vi "Meca_Jocobian.vi"(0 "Joints":sgl[](array[numeric]), 1 "TRF_XYZ":sgl[](array[numeric])) -> (2 "J":dbl[][](array[numeric]), 3 "J-":dbl[][](array[numeric]), 4 "JT":dbl[][](array[numeric]), 5 "J-T":dbl[][](array[numeric]))   [LabVIEW 2018]
uses:
  <vilib>/Analysis/baseanly.llb/Real Inverse Matrix.vi
  <vilib>/Analysis/Matrix/Numeric/Conversions/Matrix To Array - RM.vi
  <vilib>/Analysis/NI_AALBase.lvlib
  <vilib>/Analysis/Matrix/NI_Matrix.lvlib
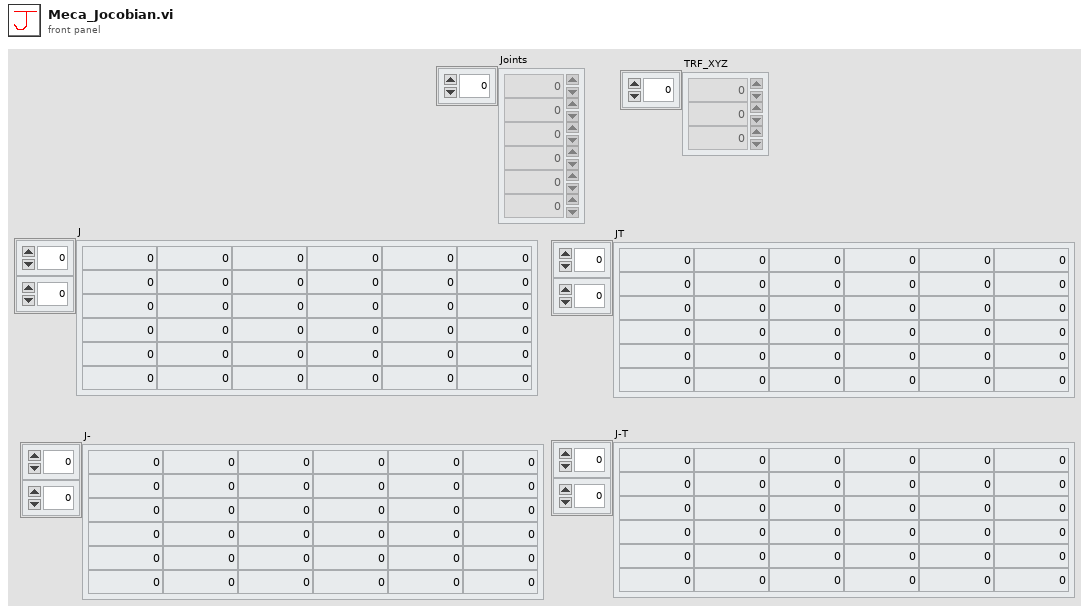
[diagram p1: front panel]
types:
  T1 = typedef "NI_Matrix.lvlib/RealMatrix.ctl" = dbl[][]
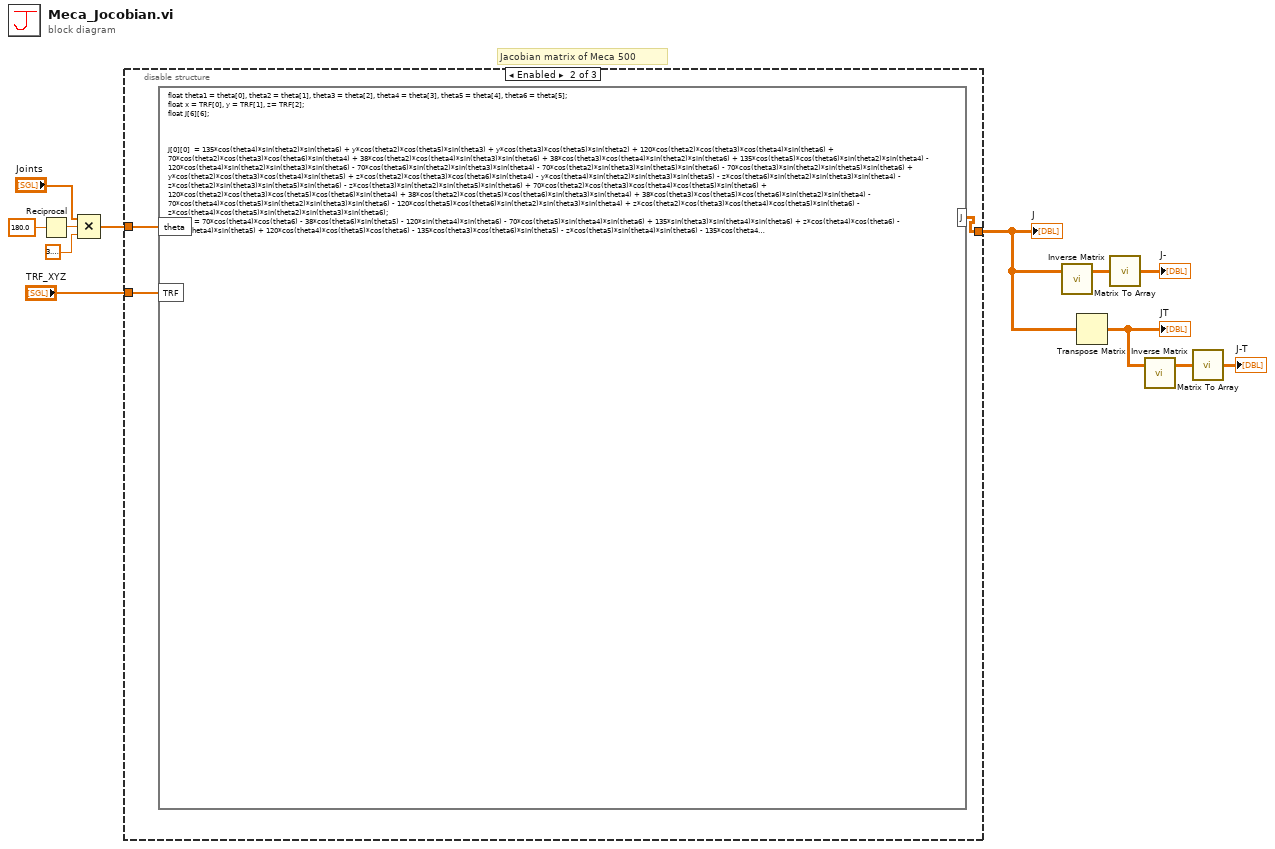
[diagram p0: block diagram]
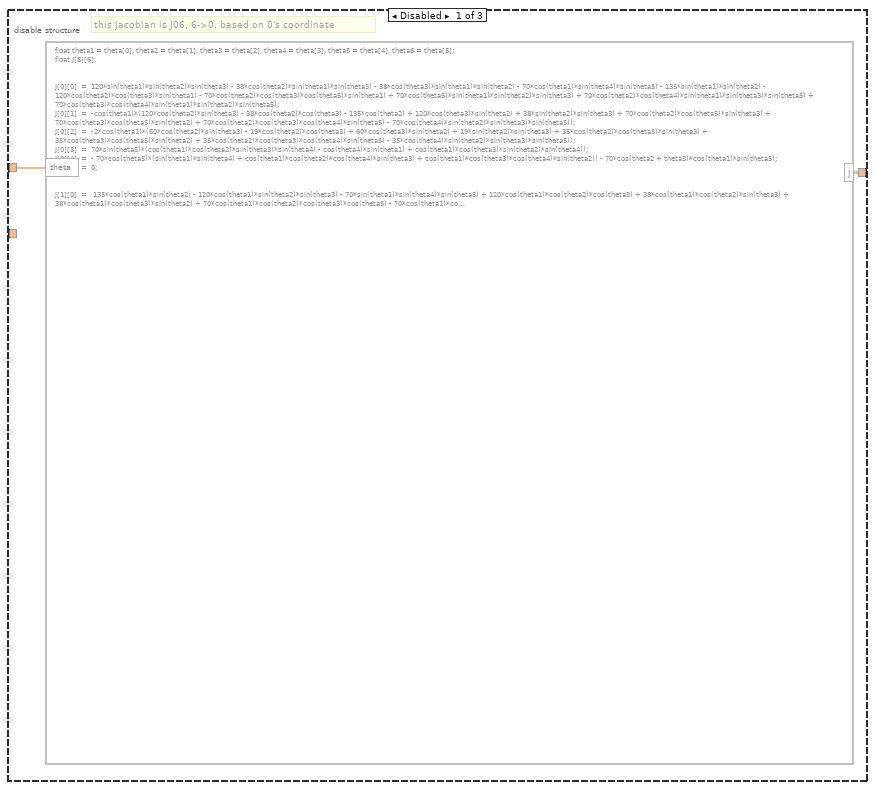
[diagram p2: hidden frame]
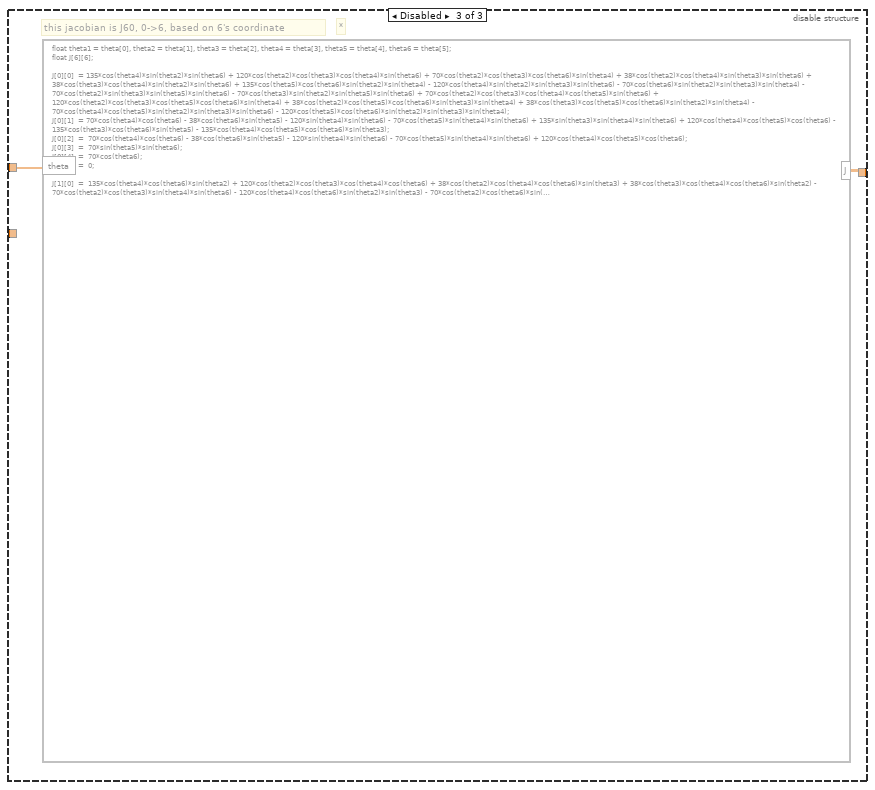
[diagram p3: hidden frame]
diagram:
  # "Jacobian matrix of Meca 500"
  n1 = Reciprocal(x=180.0 ("value")) -> (1/x=w6:dbl)
  n2 = Compound Arithmetic op=MULTIPLY("Joints", w6, 3.141592653589793) -> (w3:dbl[])
  n3 = disable-structure shown="Enabled" {
    disable-tunnel: w3 -> [w14 w16 w18]
    disable-tunnel: [w13 w15 w19] -> w8
    disable-tunnel: "TRF_XYZ" -> [_ w17 _]
    frame Disabled {
      # "this jacobian is J06, 6->0, based on 0's coordinate"
      n4 = formula code="float theta1 = theta[0], theta2 = theta[1], theta3 = theta[2], theta4 = theta[3], theta5 = theta[4], theta6 = theta[5];\nfloat J[6][6];\n\n\nJ[0][0]  =  120*sin(theta1)*sin(theta2)*sin(theta3) - 38*cos(theta2)*sin(theta1)*sin(theta3) - 38*cos(theta3)*sin(theta1)*sin(theta2) - 70*cos(theta1)*sin(theta4)*sin(theta5) - 135*sin(theta1)*sin(theta2) - 120*cos(theta2)*cos(theta3)*sin(theta1) - 70*cos(theta2)*cos(theta3)*cos(theta5)*sin(theta1) + 70*cos(theta5)*sin(theta1)*sin(theta2)*sin(theta3) + 70*cos(theta2)*cos(theta4)*sin(theta1)*sin(theta3)*sin(theta5) + 70*cos(theta3)*cos(theta4)*sin(theta1)*sin(theta2)*sin(theta5);\nJ[0][1]  =  -cos(theta1)*(120*cos(theta2)*sin(theta3) - 38*cos(theta2)*cos(theta3) - 135*cos(theta2) + 120*cos(theta3)*sin(theta2) + 38*sin(theta2)*sin(theta3) + 70*cos(theta2)*cos(theta5)*sin(theta3) + 70*cos(theta3)*cos(theta5)*sin(theta2) + 70*cos(theta2)*cos(theta3)*cos(theta4)*sin(theta5) - 70*cos(theta4)*sin(theta2)*sin(theta3)*sin(theta5));\nJ[0][2]  =  -2*cos(theta1)*(60*cos(theta2)*sin(theta3) - 19*cos(theta2)*cos(theta3) + 60*cos(theta3)*sin(theta2) + 19*sin(theta2)*sin(theta3) + 35*cos(theta2)*cos(theta5)*sin(theta3) + 35*cos(theta3)*cos(theta5)*sin(theta2) + 35*cos(theta2)*cos(theta3)*cos(theta4)*sin(theta5) - 35*cos(theta4)*sin(theta2)*sin(theta3)*sin(theta5));\nJ[0][3]  =  70*sin(theta5)*(cos(theta1)*cos(theta2)*sin(theta3)*sin(theta4) - cos(theta4)*sin(theta1) + cos(theta1)*cos(theta3)*sin(theta2)*sin(theta4));\nJ[0][4]  =  - 70*cos(theta5)*(sin(theta1)*sin(theta4) + cos(theta1)*cos(theta2)*cos(theta4)*sin(theta3) + cos(theta1)*cos(theta3)*cos(theta4)*sin(theta2)) - 70*cos(theta2 + theta3)*cos(theta1)*sin(theta5);\nJ[0][5]  =  0;\n\n\nJ[1][0]  =  \t135*cos(theta1)*sin(theta2) - 120*cos(theta1)*sin(theta2)*sin(theta3) - 70*sin(theta1)*sin(theta4)*sin(theta5) + 120*cos(theta1)*cos(theta2)*cos(theta3) + 38*cos(theta1)*cos(theta2)*sin(theta3) + 38*cos(theta1)*cos(theta3)*sin(theta2) + 70*cos(theta1)*cos(theta2)*cos(theta3)*cos(theta5) - 70*cos(theta1)*cos(theta5)*sin(theta2)*sin(theta3) - 70*cos(theta1)*cos(theta2)*cos(theta4)*sin(theta3)*sin(theta5) - 70*cos(theta1)*cos(theta3)*cos(theta4)*sin(theta2)*sin(theta5);\nJ[1][1]  =  -sin(theta1)*(120*cos(theta2)*sin(theta3) - 38*cos(theta2)*cos(theta3) - 135*cos(theta2) + 120*cos(theta3)*sin(theta2) + 38*sin(theta2)*sin(theta3) + 70*cos(theta2)*cos(theta5)*sin(theta3) + 70*cos(theta3)*cos(theta5)*sin(theta2) + 70*cos(theta2)*cos(theta3)*cos(theta4)*sin(theta5) - 70*cos(theta4)*sin(theta2)*sin(theta3)*sin(theta5));\nJ[1][2]  =  -2*sin(theta1)*(60*cos(theta2)*sin(theta3) - 19*cos(theta2)*cos(theta3) + 60*cos(theta3)*sin(theta2) + 19*sin(theta2)*sin(theta3) + 35*cos(theta2)*cos(theta5)*sin(theta3) + 35*cos(theta3)*cos(theta5)*sin(theta2) + 35*cos(theta2)*cos(theta3)*cos(theta4)*sin(theta5) - 35*cos(theta4)*sin(theta2)*sin(theta3)*sin(theta5));\nJ[1][3]  =  70*sin(theta5)*(cos(theta1)*cos(theta4) + cos(theta2)*sin(theta1)*sin(theta3)*sin(theta4) + cos(theta3)*sin(theta1)*sin(theta2)*sin(theta4));\nJ[1][4]  =  - 70*cos(theta5)*(cos(theta2)*cos(theta4)*sin(theta1)*sin(theta3) - cos(theta1)*sin(theta4) + cos(theta3)*cos(theta4)*sin(theta1)*sin(theta2)) - 70*cos(theta2 + theta3)*sin(theta1)*sin(theta5);\nJ[1][5]  =  0;\n\nJ[2][0]  =  0;\nJ[2][1]  = \t120*sin(theta2)*sin(theta3) - 120*cos(theta2)*cos(theta3) - 38*cos(theta2)*sin(theta3) - 38*cos(theta3)*sin(theta2) - 135*sin(theta2) + 70*cos(theta5)*sin(theta2)*sin(theta3) - 70*cos(theta2)*cos(theta3)*cos(theta5) + 70*cos(theta2)*cos(theta4)*sin(theta3)*sin(theta5) + 70*cos(theta3)*cos(theta4)*sin(theta2)*sin(theta5);\nJ[2][2]  = \t120*sin(theta2)*sin(theta3) - 38*cos(theta2)*sin(theta3) - 38*cos(theta3)*sin(theta2) - 120*cos(theta2)*cos(theta3) + 70*cos(theta5)*sin(theta2)*sin(theta3) - 70*cos(theta2)*cos(theta3)*cos(theta5) + 70*cos(theta2)*cos(theta4)*sin(theta3)*sin(theta5) + 70*cos(theta3)*cos(theta4)*sin(theta2)*sin(theta5);\nJ[2][3]  = \t70*cos(theta2 + theta3)*sin(theta4)*sin(theta5);\nJ[2][4]  = \t70*sin(theta2 + theta3)*sin(theta5) - 70*cos(theta2 + theta3)*cos(theta4)*cos(theta5);\nJ[2][5]  = \t0;\n\nJ[3][0]  = theta4*sin(theta1)*sin(theta2)*sin(theta3) - theta3*cos(theta1) - theta5*cos(theta1)*cos(theta4) - theta4*cos(theta2)*cos(theta3)*sin(theta1) - theta6*cos(theta1)*sin(theta4)*sin(theta5) - theta2*cos(theta1) - theta6*cos(theta2)*cos(theta3)*cos(theta5)*sin(theta1) - theta5*cos(theta2)*sin(theta1)*sin(theta3)*sin(theta4) - theta5*cos(theta3)*sin(theta1)*sin(theta2)*sin(theta4) + theta6*cos(theta5)*sin(theta1)*sin(theta2)*sin(theta3) + theta6*cos(theta2)*cos(theta4)*sin(theta1)*sin(theta3)*sin(theta5) + theta6*cos(theta3)*cos(theta4)*sin(theta1)*sin(theta2)*sin(theta5);\nJ[3][1]  = theta5*cos(theta1)*cos(theta2)*cos(theta3)*sin(theta4) - theta4*cos(theta1)*cos(theta2)*sin(theta3) - theta4*cos(theta1)*cos(theta3)*sin(theta2) - sin(theta1) - theta6*cos(theta1)*cos(theta2)*cos(theta5)*sin(theta3) - theta6*cos(theta1)*cos(theta3)*cos(theta5)*sin(theta2) - theta5*cos(theta1)*sin(theta2)*sin(theta3)*sin(theta4) - theta6*cos(theta1)*cos(theta2)*cos(theta3)*cos(theta4)*sin(theta5) + theta6*cos(theta1)*cos(theta4)*sin(theta2)*sin(theta3)*sin(theta5);\nJ[3][2]  = theta5*cos(theta1)*cos(theta2)*cos(theta3)*sin(theta4) - theta4*cos(theta1)*cos(theta2)*sin(theta3) - theta4*cos(theta1)*cos(theta3)*sin(theta2) - sin(theta1) - theta6*cos(theta1)*cos(theta2)*cos(theta5)*sin(theta3) - theta6*cos(theta1)*cos(theta3)*cos(theta5)*sin(theta2) - theta5*cos(theta1)*sin(theta2)*sin(theta3)*sin(theta4) - theta6*cos(theta1)*cos(theta2)*cos(theta3)*cos(theta4)*sin(theta5) + theta6*cos(theta1)*cos(theta4)*sin(theta2)*sin(theta3)*sin(theta5);\nJ[3][3]  = theta5*(sin(theta1)*sin(theta4) + cos(theta1)*cos(theta2)*cos(theta4)*sin(theta3) + cos(theta1)*cos(theta3)*cos(theta4)*sin(theta2)) - cos(theta1)*sin(theta2)*sin(theta3) + cos(theta1)*cos(theta2)*cos(theta3) + theta6*sin(theta5)*(cos(theta1)*cos(theta2)*sin(theta3)*sin(theta4) - cos(theta4)*sin(theta1) + cos(theta1)*cos(theta3)*sin(theta2)*sin(theta4));\nJ[3][4]  = - cos(theta4)*sin(theta1) - theta6*(cos(theta5)*(sin(theta1)*sin(theta4) - cos(theta4)*(cos(theta1)*sin(theta3)*sin(theta2 - pi/2) - cos(theta1)*cos(theta3)*cos(theta2 - pi/2))) - sin(theta5)*(cos(theta1)*cos(theta3)*sin(theta2 - pi/2) + cos(theta1)*cos(theta2 - pi/2)*sin(theta3))) - sin(theta4)*(cos(theta1)*sin(theta3)*sin(theta2 - pi/2) - cos(theta1)*cos(theta3)*cos(theta2 - pi/2));\nJ[3][5]  = cos(theta2 + theta3)*cos(theta1)*cos(theta5) - sin(theta5)*(sin(theta1)*sin(theta4) + cos(theta1)*cos(theta2)*cos(theta4)*sin(theta3) + cos(theta1)*cos(theta3)*cos(theta4)*sin(theta2));\n\nJ[4][0]  =\ttheta4*cos(theta1)*cos(theta2)*cos(theta3) - theta3*sin(theta1) - theta5*cos(theta4)*sin(theta1) - theta2*sin(theta1) - theta4*cos(theta1)*sin(theta2)*sin(theta3) - theta6*sin(theta1)*sin(theta4)*sin(theta5) + theta6*cos(theta1)*cos(theta2)*cos(theta3)*cos(theta5) + theta5*cos(theta1)*cos(theta2)*sin(theta3)*sin(theta4) + theta5*cos(theta1)*cos(theta3)*sin(theta2)*sin(theta4) - theta6*cos(theta1)*cos(theta5)*sin(theta2)*sin(theta3) - theta6*cos(theta1)*cos(theta2)*cos(theta4)*sin(theta3)*sin(theta5) - theta6*cos(theta1)*cos(theta3)*cos(theta4)*sin(theta2)*sin(theta5);\nJ[4][1]  =\tcos(theta1) - theta4*cos(theta2)*sin(theta1)*sin(theta3) - theta4*cos(theta3)*sin(theta1)*sin(theta2) + theta5*cos(theta2)*cos(theta3)*sin(theta1)*sin(theta4) - theta6*cos(theta2)*cos(theta5)*sin(theta1)*sin(theta3) - theta6*cos(theta3)*cos(theta5)*sin(theta1)*sin(theta2) - theta5*sin(theta1)*sin(theta2)*sin(theta3)*sin(theta4) - theta6*cos(theta2)*cos(theta3)*cos(theta4)*sin(theta1)*sin(theta5) + theta6*cos(theta4)*sin(theta1)*sin(theta2)*sin(theta3)*sin(theta5);\nJ[4][2]  =\tcos(theta1) - theta4*cos(theta2)*sin(theta1)*sin(theta3) - theta4*cos(theta3)*sin(theta1)*sin(theta2) + theta5*cos(theta2)*cos(theta3)*sin(theta1)*sin(theta4) - theta6*cos(theta2)*cos(theta5)*sin(theta1)*sin(theta3) - theta6*cos(theta3)*cos(theta5)*sin(theta1)*sin(theta2) - theta5*sin(theta1)*sin(theta2)*sin(theta3)*sin(theta4) - theta6*cos(theta2)*cos(theta3)*cos(theta4)*sin(theta1)*sin(theta5) + theta6*cos(theta4)*sin(theta1)*sin(theta2)*sin(theta3)*sin(theta5);\nJ[4][3]  =\ttheta5*(cos(theta2)*cos(theta4)*sin(theta1)*sin(theta3) - cos(theta1)*sin(theta4) + cos(theta3)*cos(theta4)*sin(theta1)*sin(theta2)) + theta6*sin(theta5)*(cos(theta1)*cos(theta4) + cos(theta2)*sin(theta1)*sin(theta3)*sin(theta4) + cos(theta3)*sin(theta1)*sin(theta2)*sin(theta4)) - sin(theta1)*sin(theta2)*sin(theta3) + cos(theta2)*cos(theta3)*sin(theta1);\nJ[4][4]  =\tcos(theta1)*cos(theta4) + sin(theta2 + theta3)*sin(theta1)*sin(theta4) - theta6*cos(theta2 + theta3)*sin(theta1)*sin(theta5) + theta6*cos(theta1)*cos(theta5)*sin(theta4) - theta6*cos(theta2)*cos(theta4)*cos(theta5)*sin(theta1)*sin(theta3) - theta6*cos(theta3)*cos(theta4)*cos(theta5)*sin(theta1)*sin(theta2);\nJ[4][5]  =\tcos(theta2 + theta3)*cos(theta5)*sin(theta1) - sin(theta5)*(cos(theta2)*cos(theta4)*sin(theta1)*sin(theta3) - cos(theta1)*sin(theta4) + cos(theta3)*cos(theta4)*sin(theta1)*sin(theta2));\n\nJ[5][0]  = 1;\nJ[5][1]  = theta6*sin(theta2 + theta3)*cos(theta4)*sin(theta5) - theta6*cos(theta2 + theta3)*cos(theta5) - theta5*sin(theta2 + theta3)*sin(theta4) - theta4*cos(theta2 + theta3);\nJ[5][2]  = theta6*sin(theta2 + theta3)*cos(theta4)*sin(theta5) - theta6*cos(theta2 + theta3)*cos(theta5) - theta5*sin(theta2 + theta3)*sin(theta4) - theta4*cos(theta2 + theta3);\nJ[5][3]  = theta5*cos(theta2)*cos(theta3)*cos(theta4) - cos(theta3)*sin(theta2) - cos(theta2)*sin(theta3) - theta5*cos(theta4)*sin(theta2)*sin(theta3) + theta6*cos(theta2)*cos(theta3)*sin(theta4)*sin(theta5) - theta6*sin(theta2)*sin(theta3)*sin(theta4)*sin(theta5);\nJ[5][4]  = theta6*(sin(theta2 + theta3)*sin(theta5) - cos(theta2 + theta3)*cos(theta4)*cos(theta5)) + cos(theta2 + theta3)*sin(theta4);\nJ[5][5]  = - sin(theta2 + theta3)*cos(theta5) - cos(theta2 + theta3)*cos(theta4)*sin(theta5);"("theta"=w14) -> ("J"=w13:dbl[][])
    }
    frame Enabled {
      n5 = formula code="float theta1 = theta[0], theta2 = theta[1], theta3 = theta[2], theta4 = theta[3], theta5 = theta[4], theta6 = theta[5];\nfloat x = TRF[0], y = TRF[1], z= TRF[2];\nfloat J[6][6];\n\n\n\nJ[0][0]  = 135*cos(theta4)*sin(theta2)*sin(theta6) + y*cos(theta2)*cos(theta5)*sin(theta3) + y*cos(theta3)*cos(theta5)*sin(theta2) + 120*cos(theta2)*cos(theta3)*cos(theta4)*sin(theta6) + 70*cos(theta2)*cos(theta3)*cos(theta6)*sin(theta4) + 38*cos(theta2)*cos(theta4)*sin(theta3)*sin(theta6) + 38*cos(theta3)*cos(theta4)*sin(theta2)*sin(theta6) + 135*cos(theta5)*cos(theta6)*sin(theta2)*sin(theta4) - 120*cos(theta4)*sin(theta2)*sin(theta3)*sin(theta6) - 70*cos(theta6)*sin(theta2)*sin(theta3)*sin(theta4) - 70*cos(theta2)*sin(theta3)*sin(theta5)*sin(theta6) - 70*cos(theta3)*sin(theta2)*sin(theta5)*sin(theta6) + y*cos(theta2)*cos(theta3)*cos(theta4)*sin(theta5) + z*cos(theta2)*cos(theta3)*cos(theta6)*sin(theta4) - y*cos(theta4)*sin(theta2)*sin(theta3)*sin(theta5) - z*cos(theta6)*sin(theta2)*sin(theta3)*sin(theta4) - z*cos(theta2)*sin(theta3)*sin(theta5)*sin(theta6) - z*cos(theta3)*sin(theta2)*sin(theta5)*sin(theta6) + 70*cos(theta2)*cos(theta3)*cos(theta4)*cos(theta5)*sin(theta6) + 120*cos(theta2)*cos(theta3)*cos(theta5)*cos(theta6)*sin(theta4) + 38*cos(theta2)*cos(theta5)*cos(theta6)*sin(theta3)*sin(theta4) + 38*cos(theta3)*cos(theta5)*cos(theta6)*sin(theta2)*sin(theta4) - 70*cos(theta4)*cos(theta5)*sin(theta2)*sin(theta3)*sin(theta6) - 120*cos(theta5)*cos(theta6)*sin(theta2)*sin(theta3)*sin(theta4) + z*cos(theta2)*cos(theta3)*cos(theta4)*cos(theta5)*sin(theta6) - z*cos(theta4)*cos(theta5)*sin(theta2)*sin(theta3)*sin(theta6); \nJ[0][1]  = 70*cos(theta4)*cos(theta6) - 38*cos(theta6)*sin(theta5) - 120*sin(theta4)*sin(theta6) - 70*cos(theta5)*sin(theta4)*sin(theta6) + 135*sin(theta3)*sin(theta4)*sin(theta6) + z*cos(theta4)*cos(theta6) - y*sin(theta4)*sin(theta5) + 120*cos(theta4)*cos(theta5)*cos(theta6) - 135*cos(theta3)*cos(theta6)*sin(theta5) - z*cos(theta5)*sin(theta4)*sin(theta6) - 135*cos(theta4)*cos(theta5)*cos(theta6)*sin(theta3);\nJ[0][2]  = 70*cos(theta4)*cos(theta6) - 38*cos(theta6)*sin(theta5) - 120*sin(theta4)*sin(theta6) - 70*cos(theta5)*sin(theta4)*sin(theta6) + z*cos(theta4)*cos(theta6) - y*sin(theta4)*sin(theta5) + 120*cos(theta4)*cos(theta5)*cos(theta6) - z*cos(theta5)*sin(theta4)*sin(theta6);                    \nJ[0][3]  = 70*sin(theta5)*sin(theta6) - y*cos(theta5) + z*sin(theta5)*sin(theta6);             \nJ[0][4]  = cos(theta6)*(z + 70); \nJ[0][5]  = -y;\n\nJ[1][0]  = 135*cos(theta4)*cos(theta6)*sin(theta2) - x*cos(theta2)*cos(theta5)*sin(theta3) - x*cos(theta3)*cos(theta5)*sin(theta2) + 120*cos(theta2)*cos(theta3)*cos(theta4)*cos(theta6) + 38*cos(theta2)*cos(theta4)*cos(theta6)*sin(theta3) + 38*cos(theta3)*cos(theta4)*cos(theta6)*sin(theta2) - 70*cos(theta2)*cos(theta3)*sin(theta4)*sin(theta6) - 120*cos(theta4)*cos(theta6)*sin(theta2)*sin(theta3) - 70*cos(theta2)*cos(theta6)*sin(theta3)*sin(theta5) - 70*cos(theta3)*cos(theta6)*sin(theta2)*sin(theta5) - 135*cos(theta5)*sin(theta2)*sin(theta4)*sin(theta6) + 70*sin(theta2)*sin(theta3)*sin(theta4)*sin(theta6) - x*cos(theta2)*cos(theta3)*cos(theta4)*sin(theta5) - z*cos(theta2)*cos(theta3)*sin(theta4)*sin(theta6) - z*cos(theta2)*cos(theta6)*sin(theta3)*sin(theta5) - z*cos(theta3)*cos(theta6)*sin(theta2)*sin(theta5) + x*cos(theta4)*sin(theta2)*sin(theta3)*sin(theta5) + z*sin(theta2)*sin(theta3)*sin(theta4)*sin(theta6) + 70*cos(theta2)*cos(theta3)*cos(theta4)*cos(theta5)*cos(theta6) - 120*cos(theta2)*cos(theta3)*cos(theta5)*sin(theta4)*sin(theta6) - 70*cos(theta4)*cos(theta5)*cos(theta6)*sin(theta2)*sin(theta3) - 38*cos(theta2)*cos(theta5)*sin(theta3)*sin(theta4)*sin(theta6) - 38*cos(theta3)*cos(theta5)*sin(theta2)*sin(theta4)*sin(theta6) + 120*cos(theta5)*sin(theta2)*sin(theta3)*sin(theta4)*sin(theta6) + z*cos(theta2)*cos(theta3)*cos(theta4)*cos(theta5)*cos(theta6) - z*cos(theta4)*cos(theta5)*cos(theta6)*sin(theta2)*sin(theta3); \nJ[1][1]  = 38*sin(theta5)*sin(theta6) - 120*cos(theta6)*sin(theta4) - 70*cos(theta4)*sin(theta6) + 135*cos(theta6)*sin(theta3)*sin(theta4) + 135*cos(theta3)*sin(theta5)*sin(theta6) - z*cos(theta4)*sin(theta6) + x*sin(theta4)*sin(theta5) - 120*cos(theta4)*cos(theta5)*sin(theta6) - 70*cos(theta5)*cos(theta6)*sin(theta4) - z*cos(theta5)*cos(theta6)*sin(theta4) + 135*cos(theta4)*cos(theta5)*sin(theta3)*sin(theta6); \nJ[1][2]  = 38*sin(theta5)*sin(theta6) - 120*cos(theta6)*sin(theta4) - 70*cos(theta4)*sin(theta6) - z*cos(theta4)*sin(theta6) + x*sin(theta4)*sin(theta5) - 120*cos(theta4)*cos(theta5)*sin(theta6) - 70*cos(theta5)*cos(theta6)*sin(theta4) - z*cos(theta5)*cos(theta6)*sin(theta4);                    \nJ[1][3]  = 70*cos(theta6)*sin(theta5) + x*cos(theta5) + z*cos(theta6)*sin(theta5);            \nJ[1][4]  = -sin(theta6)*(z + 70);  \nJ[1][5]  = x;\n\n\nJ[2][0]  = 135*sin(theta2)*sin(theta4)*sin(theta5) + 120*cos(theta2)*cos(theta3)*sin(theta4)*sin(theta5) + 38*cos(theta2)*sin(theta3)*sin(theta4)*sin(theta5) + 38*cos(theta3)*sin(theta2)*sin(theta4)*sin(theta5) - 120*sin(theta2)*sin(theta3)*sin(theta4)*sin(theta5) - x*cos(theta2)*cos(theta3)*cos(theta6)*sin(theta4) + y*cos(theta2)*cos(theta3)*sin(theta4)*sin(theta6) + y*cos(theta2)*cos(theta6)*sin(theta3)*sin(theta5) + y*cos(theta3)*cos(theta6)*sin(theta2)*sin(theta5) + x*cos(theta6)*sin(theta2)*sin(theta3)*sin(theta4) + x*cos(theta2)*sin(theta3)*sin(theta5)*sin(theta6) + x*cos(theta3)*sin(theta2)*sin(theta5)*sin(theta6) - y*sin(theta2)*sin(theta3)*sin(theta4)*sin(theta6) - y*cos(theta2)*cos(theta3)*cos(theta4)*cos(theta5)*cos(theta6) - x*cos(theta2)*cos(theta3)*cos(theta4)*cos(theta5)*sin(theta6) + y*cos(theta4)*cos(theta5)*cos(theta6)*sin(theta2)*sin(theta3) + x*cos(theta4)*cos(theta5)*sin(theta2)*sin(theta3)*sin(theta6); \nJ[2][1]  = 38*cos(theta5) + 135*cos(theta3)*cos(theta5) + 120*cos(theta4)*sin(theta5) - 135*cos(theta4)*sin(theta3)*sin(theta5) - x*cos(theta4)*cos(theta6) + y*cos(theta4)*sin(theta6) + y*cos(theta5)*cos(theta6)*sin(theta4) + x*cos(theta5)*sin(theta4)*sin(theta6);  \nJ[2][2]  = 38*cos(theta5) + 120*cos(theta4)*sin(theta5) - x*cos(theta4)*cos(theta6) + y*cos(theta4)*sin(theta6) + y*cos(theta5)*cos(theta6)*sin(theta4) + x*cos(theta5)*sin(theta4)*sin(theta6);\nJ[2][3]  = -sin(theta5)*(y*cos(theta6) + x*sin(theta6));\nJ[2][4]  = y*sin(theta6) - x*cos(theta6);\nJ[2][5]  = 0;\n\nJ[3][0]  = cos(theta2)*cos(theta3)*sin(theta4)*sin(theta6) + cos(theta2)*cos(theta6)*sin(theta3)*sin(theta5) + cos(theta3)*cos(theta6)*sin(theta2)*sin(theta5) - sin(theta2)*sin(theta3)*sin(theta4)*sin(theta6) + theta2*cos(theta2)*cos(theta3)*cos(theta6)*sin(theta5) + theta3*cos(theta2)*cos(theta3)*cos(theta6)*sin(theta5) + theta4*cos(theta2)*cos(theta3)*cos(theta4)*sin(theta6) + theta5*cos(theta2)*cos(theta5)*cos(theta6)*sin(theta3) + theta5*cos(theta3)*cos(theta5)*cos(theta6)*sin(theta2) + theta6*cos(theta2)*cos(theta3)*cos(theta6)*sin(theta4) - theta2*cos(theta2)*sin(theta3)*sin(theta4)*sin(theta6) - theta2*cos(theta3)*sin(theta2)*sin(theta4)*sin(theta6) - theta2*cos(theta6)*sin(theta2)*sin(theta3)*sin(theta5) - theta3*cos(theta2)*sin(theta3)*sin(theta4)*sin(theta6) - theta3*cos(theta3)*sin(theta2)*sin(theta4)*sin(theta6) - theta3*cos(theta6)*sin(theta2)*sin(theta3)*sin(theta5) - theta4*cos(theta4)*sin(theta2)*sin(theta3)*sin(theta6) - theta6*cos(theta6)*sin(theta2)*sin(theta3)*sin(theta4) - theta6*cos(theta2)*sin(theta3)*sin(theta5)*sin(theta6) - theta6*cos(theta3)*sin(theta2)*sin(theta5)*sin(theta6) - cos(theta2)*cos(theta3)*cos(theta4)*cos(theta5)*cos(theta6) + cos(theta4)*cos(theta5)*cos(theta6)*sin(theta2)*sin(theta3) + theta2*cos(theta2)*cos(theta4)*cos(theta5)*cos(theta6)*sin(theta3) + theta2*cos(theta3)*cos(theta4)*cos(theta5)*cos(theta6)*sin(theta2) + theta3*cos(theta2)*cos(theta4)*cos(theta5)*cos(theta6)*sin(theta3) + theta3*cos(theta3)*cos(theta4)*cos(theta5)*cos(theta6)*sin(theta2) + theta4*cos(theta2)*cos(theta3)*cos(theta5)*cos(theta6)*sin(theta4) + theta5*cos(theta2)*cos(theta3)*cos(theta4)*cos(theta6)*sin(theta5) + theta6*cos(theta2)*cos(theta3)*cos(theta4)*cos(theta5)*sin(theta6) - theta4*cos(theta5)*cos(theta6)*sin(theta2)*sin(theta3)*sin(theta4) - theta5*cos(theta4)*cos(theta6)*sin(theta2)*sin(theta3)*sin(theta5) - theta6*cos(theta4)*cos(theta5)*sin(theta2)*sin(theta3)*sin(theta6);\nJ[3][1]  = cos(theta4)*sin(theta6) + theta6*cos(theta4)*cos(theta6) - theta4*sin(theta4)*sin(theta6) + cos(theta5)*cos(theta6)*sin(theta4) + theta4*cos(theta4)*cos(theta5)*cos(theta6) - theta5*cos(theta6)*sin(theta4)*sin(theta5) - theta6*cos(theta5)*sin(theta4)*sin(theta6);   \nJ[3][2]  = cos(theta4)*sin(theta6) + theta6*cos(theta4)*cos(theta6) - theta4*sin(theta4)*sin(theta6) + cos(theta5)*cos(theta6)*sin(theta4) + theta4*cos(theta4)*cos(theta5)*cos(theta6) - theta5*cos(theta6)*sin(theta4)*sin(theta5) - theta6*cos(theta5)*sin(theta4)*sin(theta6); \nJ[3][3]  = theta6*sin(theta5)*sin(theta6) - theta5*cos(theta5)*cos(theta6) - cos(theta6)*sin(theta5); \nJ[3][4]  = sin(theta6) + theta6*cos(theta6);  \nJ[3][5]  = 0;\n\nJ[4][0]  = cos(theta2)*cos(theta3)*cos(theta6)*sin(theta4) - cos(theta6)*sin(theta2)*sin(theta3)*sin(theta4) - cos(theta2)*sin(theta3)*sin(theta5)*sin(theta6) - cos(theta3)*sin(theta2)*sin(theta5)*sin(theta6) + theta4*cos(theta2)*cos(theta3)*cos(theta4)*cos(theta6) - theta2*cos(theta2)*cos(theta6)*sin(theta3)*sin(theta4) - theta2*cos(theta3)*cos(theta6)*sin(theta2)*sin(theta4) - theta2*cos(theta2)*cos(theta3)*sin(theta5)*sin(theta6) - theta3*cos(theta2)*cos(theta6)*sin(theta3)*sin(theta4) - theta3*cos(theta3)*cos(theta6)*sin(theta2)*sin(theta4) - theta3*cos(theta2)*cos(theta3)*sin(theta5)*sin(theta6) - theta4*cos(theta4)*cos(theta6)*sin(theta2)*sin(theta3) - theta5*cos(theta2)*cos(theta5)*sin(theta3)*sin(theta6) - theta5*cos(theta3)*cos(theta5)*sin(theta2)*sin(theta6) - theta6*cos(theta2)*cos(theta3)*sin(theta4)*sin(theta6) - theta6*cos(theta2)*cos(theta6)*sin(theta3)*sin(theta5) - theta6*cos(theta3)*cos(theta6)*sin(theta2)*sin(theta5) + theta2*sin(theta2)*sin(theta3)*sin(theta5)*sin(theta6) + theta3*sin(theta2)*sin(theta3)*sin(theta5)*sin(theta6) + theta6*sin(theta2)*sin(theta3)*sin(theta4)*sin(theta6) + cos(theta2)*cos(theta3)*cos(theta4)*cos(theta5)*sin(theta6) - cos(theta4)*cos(theta5)*sin(theta2)*sin(theta3)*sin(theta6) + theta6*cos(theta2)*cos(theta3)*cos(theta4)*cos(theta5)*cos(theta6) - theta2*cos(theta2)*cos(theta4)*cos(theta5)*sin(theta3)*sin(theta6) - theta2*cos(theta3)*cos(theta4)*cos(theta5)*sin(theta2)*sin(theta6) - theta3*cos(theta2)*cos(theta4)*cos(theta5)*sin(theta3)*sin(theta6) - theta3*cos(theta3)*cos(theta4)*cos(theta5)*sin(theta2)*sin(theta6) - theta4*cos(theta2)*cos(theta3)*cos(theta5)*sin(theta4)*sin(theta6) - theta5*cos(theta2)*cos(theta3)*cos(theta4)*sin(theta5)*sin(theta6) - theta6*cos(theta4)*cos(theta5)*cos(theta6)*sin(theta2)*sin(theta3) + theta4*cos(theta5)*sin(theta2)*sin(theta3)*sin(theta4)*sin(theta6) + theta5*cos(theta4)*sin(theta2)*sin(theta3)*sin(theta5)*sin(theta6);\nJ[4][1]  = cos(theta4)*cos(theta6) - cos(theta5)*sin(theta4)*sin(theta6) - theta4*cos(theta6)*sin(theta4) - theta6*cos(theta4)*sin(theta6) - theta4*cos(theta4)*cos(theta5)*sin(theta6) - theta6*cos(theta5)*cos(theta6)*sin(theta4) + theta5*sin(theta4)*sin(theta5)*sin(theta6);   \nJ[4][2]  = cos(theta4)*cos(theta6) - cos(theta5)*sin(theta4)*sin(theta6) - theta4*cos(theta6)*sin(theta4) - theta6*cos(theta4)*sin(theta6) - theta4*cos(theta4)*cos(theta5)*sin(theta6) - theta6*cos(theta5)*cos(theta6)*sin(theta4) + theta5*sin(theta4)*sin(theta5)*sin(theta6); \nJ[4][3]  = sin(theta5)*sin(theta6) + theta5*cos(theta5)*sin(theta6) + theta6*cos(theta6)*sin(theta5); \nJ[4][4]  = cos(theta6) - theta6*sin(theta6);  \nJ[4][5]  = 0;\n\nJ[5][0]  = theta2*cos(theta5)*sin(theta2)*sin(theta3) - cos(theta3)*cos(theta5)*sin(theta2) - theta2*cos(theta2)*cos(theta3)*cos(theta5) - theta3*cos(theta2)*cos(theta3)*cos(theta5) - cos(theta2)*cos(theta5)*sin(theta3) + theta3*cos(theta5)*sin(theta2)*sin(theta3) + theta5*cos(theta2)*sin(theta3)*sin(theta5) + theta5*cos(theta3)*sin(theta2)*sin(theta5) - cos(theta2)*cos(theta3)*cos(theta4)*sin(theta5) + cos(theta4)*sin(theta2)*sin(theta3)*sin(theta5) - theta5*cos(theta2)*cos(theta3)*cos(theta4)*cos(theta5) + theta2*cos(theta2)*cos(theta4)*sin(theta3)*sin(theta5) + theta2*cos(theta3)*cos(theta4)*sin(theta2)*sin(theta5) + theta3*cos(theta2)*cos(theta4)*sin(theta3)*sin(theta5) + theta3*cos(theta3)*cos(theta4)*sin(theta2)*sin(theta5) + theta4*cos(theta2)*cos(theta3)*sin(theta4)*sin(theta5) + theta5*cos(theta4)*cos(theta5)*sin(theta2)*sin(theta3) - theta4*sin(theta2)*sin(theta3)*sin(theta4)*sin(theta5);\nJ[5][1]  =  sin(theta4)*sin(theta5) + theta4*cos(theta4)*sin(theta5) + theta5*cos(theta5)*sin(theta4);\nJ[5][2]  = sin(theta4)*sin(theta5) + theta4*cos(theta4)*sin(theta5) + theta5*cos(theta5)*sin(theta4);                                                          \nJ[5][3]  = cos(theta5) - theta5*sin(theta5);                                \nJ[5][4]  = 0;  \nJ[5][5]  = 1;"("theta"=w16, "TRF"=w17) -> ("J"=w15:dbl[][])
    }
    frame Disabled {
      # "*"
      # "this jacobian is J60, 0->6, based on 6's coordinate"
      n6 = formula code="float theta1 = theta[0], theta2 = theta[1], theta3 = theta[2], theta4 = theta[3], theta5 = theta[4], theta6 = theta[5];\nfloat J[6][6];\n\nJ[0][0]  = 135*cos(theta4)*sin(theta2)*sin(theta6) + 120*cos(theta2)*cos(theta3)*cos(theta4)*sin(theta6) + 70*cos(theta2)*cos(theta3)*cos(theta6)*sin(theta4) + 38*cos(theta2)*cos(theta4)*sin(theta3)*sin(theta6) + 38*cos(theta3)*cos(theta4)*sin(theta2)*sin(theta6) + 135*cos(theta5)*cos(theta6)*sin(theta2)*sin(theta4) - 120*cos(theta4)*sin(theta2)*sin(theta3)*sin(theta6) - 70*cos(theta6)*sin(theta2)*sin(theta3)*sin(theta4) - 70*cos(theta2)*sin(theta3)*sin(theta5)*sin(theta6) - 70*cos(theta3)*sin(theta2)*sin(theta5)*sin(theta6) + 70*cos(theta2)*cos(theta3)*cos(theta4)*cos(theta5)*sin(theta6) + 120*cos(theta2)*cos(theta3)*cos(theta5)*cos(theta6)*sin(theta4) + 38*cos(theta2)*cos(theta5)*cos(theta6)*sin(theta3)*sin(theta4) + 38*cos(theta3)*cos(theta5)*cos(theta6)*sin(theta2)*sin(theta4) - 70*cos(theta4)*cos(theta5)*sin(theta2)*sin(theta3)*sin(theta6) - 120*cos(theta5)*cos(theta6)*sin(theta2)*sin(theta3)*sin(theta4);\nJ[0][1]  = 70*cos(theta4)*cos(theta6) - 38*cos(theta6)*sin(theta5) - 120*sin(theta4)*sin(theta6) - 70*cos(theta5)*sin(theta4)*sin(theta6) + 135*sin(theta3)*sin(theta4)*sin(theta6) + 120*cos(theta4)*cos(theta5)*cos(theta6) - 135*cos(theta3)*cos(theta6)*sin(theta5) - 135*cos(theta4)*cos(theta5)*cos(theta6)*sin(theta3);   \nJ[0][2]  =  70*cos(theta4)*cos(theta6) - 38*cos(theta6)*sin(theta5) - 120*sin(theta4)*sin(theta6) - 70*cos(theta5)*sin(theta4)*sin(theta6) + 120*cos(theta4)*cos(theta5)*cos(theta6);\nJ[0][3]  =  70*sin(theta5)*sin(theta6);\nJ[0][4]  =  70*cos(theta6);\nJ[0][5]  = \t0;\n\nJ[1][0]  = \t135*cos(theta4)*cos(theta6)*sin(theta2) + 120*cos(theta2)*cos(theta3)*cos(theta4)*cos(theta6) + 38*cos(theta2)*cos(theta4)*cos(theta6)*sin(theta3) + 38*cos(theta3)*cos(theta4)*cos(theta6)*sin(theta2) - 70*cos(theta2)*cos(theta3)*sin(theta4)*sin(theta6) - 120*cos(theta4)*cos(theta6)*sin(theta2)*sin(theta3) - 70*cos(theta2)*cos(theta6)*sin(theta3)*sin(theta5) - 70*cos(theta3)*cos(theta6)*sin(theta2)*sin(theta5) - 135*cos(theta5)*sin(theta2)*sin(theta4)*sin(theta6) + 70*sin(theta2)*sin(theta3)*sin(theta4)*sin(theta6) + 70*cos(theta2)*cos(theta3)*cos(theta4)*cos(theta5)*cos(theta6) - 120*cos(theta2)*cos(theta3)*cos(theta5)*sin(theta4)*sin(theta6) - 70*cos(theta4)*cos(theta5)*cos(theta6)*sin(theta2)*sin(theta3) - 38*cos(theta2)*cos(theta5)*sin(theta3)*sin(theta4)*sin(theta6) - 38*cos(theta3)*cos(theta5)*sin(theta2)*sin(theta4)*sin(theta6) + 120*cos(theta5)*sin(theta2)*sin(theta3)*sin(theta4)*sin(theta6);\nJ[1][1]  =  38*sin(theta5)*sin(theta6) - 120*cos(theta6)*sin(theta4) - 70*cos(theta4)*sin(theta6) + 135*cos(theta6)*sin(theta3)*sin(theta4) + 135*cos(theta3)*sin(theta5)*sin(theta6) - 120*cos(theta4)*cos(theta5)*sin(theta6) - 70*cos(theta5)*cos(theta6)*sin(theta4) + 135*cos(theta4)*cos(theta5)*sin(theta3)*sin(theta6);\nJ[1][2]  = 38*sin(theta5)*sin(theta6) - 120*cos(theta6)*sin(theta4) - 70*cos(theta4)*sin(theta6) - 120*cos(theta4)*cos(theta5)*sin(theta6) - 70*cos(theta5)*cos(theta6)*sin(theta4);\nJ[1][3]  =  70*cos(theta6)*sin(theta5);\nJ[1][4]  = -70*sin(theta6);\nJ[1][5]  = \t0;\n\nJ[2][0]  =  sin(theta4)*sin(theta5)*(135*sin(theta2) + 2*sqrt(3961)*cos(theta2 + theta3 - atan(19/60)));\nJ[2][1]  =  38*cos(theta5) + 135*cos(theta3)*cos(theta5) + 120*cos(theta4)*sin(theta5) - 135*cos(theta4)*sin(theta3)*sin(theta5);\nJ[2][2]  = \t38*cos(theta5) + 120*cos(theta4)*sin(theta5);\nJ[2][3]  = 0;\nJ[2][4]  = 0;\nJ[2][5]  = 0;\n\nJ[3][0]  = cos(theta2)*cos(theta3)*sin(theta4)*sin(theta6) + cos(theta2)*cos(theta6)*sin(theta3)*sin(theta5) + cos(theta3)*cos(theta6)*sin(theta2)*sin(theta5) - sin(theta2)*sin(theta3)*sin(theta4)*sin(theta6) + theta2*cos(theta2)*cos(theta3)*cos(theta6)*sin(theta5) + theta3*cos(theta2)*cos(theta3)*cos(theta6)*sin(theta5) + theta4*cos(theta2)*cos(theta3)*cos(theta4)*sin(theta6) + theta5*cos(theta2)*cos(theta5)*cos(theta6)*sin(theta3) + theta5*cos(theta3)*cos(theta5)*cos(theta6)*sin(theta2) + theta6*cos(theta2)*cos(theta3)*cos(theta6)*sin(theta4) - theta2*cos(theta2)*sin(theta3)*sin(theta4)*sin(theta6) - theta2*cos(theta3)*sin(theta2)*sin(theta4)*sin(theta6) - theta2*cos(theta6)*sin(theta2)*sin(theta3)*sin(theta5) - theta3*cos(theta2)*sin(theta3)*sin(theta4)*sin(theta6) - theta3*cos(theta3)*sin(theta2)*sin(theta4)*sin(theta6) - theta3*cos(theta6)*sin(theta2)*sin(theta3)*sin(theta5) - theta4*cos(theta4)*sin(theta2)*sin(theta3)*sin(theta6) - theta6*cos(theta6)*sin(theta2)*sin(theta3)*sin(theta4) - theta6*cos(theta2)*sin(theta3)*sin(theta5)*sin(theta6) - theta6*cos(theta3)*sin(theta2)*sin(theta5)*sin(theta6) - cos(theta2)*cos(theta3)*cos(theta4)*cos(theta5)*cos(theta6) + cos(theta4)*cos(theta5)*cos(theta6)*sin(theta2)*sin(theta3) + theta2*cos(theta2)*cos(theta4)*cos(theta5)*cos(theta6)*sin(theta3) + theta2*cos(theta3)*cos(theta4)*cos(theta5)*cos(theta6)*sin(theta2) + theta3*cos(theta2)*cos(theta4)*cos(theta5)*cos(theta6)*sin(theta3) + theta3*cos(theta3)*cos(theta4)*cos(theta5)*cos(theta6)*sin(theta2) + theta4*cos(theta2)*cos(theta3)*cos(theta5)*cos(theta6)*sin(theta4) + theta5*cos(theta2)*cos(theta3)*cos(theta4)*cos(theta6)*sin(theta5) + theta6*cos(theta2)*cos(theta3)*cos(theta4)*cos(theta5)*sin(theta6) - theta4*cos(theta5)*cos(theta6)*sin(theta2)*sin(theta3)*sin(theta4) - theta5*cos(theta4)*cos(theta6)*sin(theta2)*sin(theta3)*sin(theta5) - theta6*cos(theta4)*cos(theta5)*sin(theta2)*sin(theta3)*sin(theta6);;\nJ[3][1]  = cos(theta4)*sin(theta6) + theta6*cos(theta4)*cos(theta6) - theta4*sin(theta4)*sin(theta6) + cos(theta5)*cos(theta6)*sin(theta4) + theta4*cos(theta4)*cos(theta5)*cos(theta6) - theta5*cos(theta6)*sin(theta4)*sin(theta5) - theta6*cos(theta5)*sin(theta4)*sin(theta6);;\nJ[3][2]  = cos(theta4)*sin(theta6) + theta6*cos(theta4)*cos(theta6) - theta4*sin(theta4)*sin(theta6) + cos(theta5)*cos(theta6)*sin(theta4) + theta4*cos(theta4)*cos(theta5)*cos(theta6) - theta5*cos(theta6)*sin(theta4)*sin(theta5) - theta6*cos(theta5)*sin(theta4)*sin(theta6);;\nJ[3][3]  = \ttheta6*sin(theta5)*sin(theta6) - theta5*cos(theta5)*cos(theta6) - cos(theta6)*sin(theta5);\nJ[3][4]  = sin(theta6) + theta6*cos(theta6);\nJ[3][5]  = \t0;\n\nJ[4][0]  = \tcos(theta2)*cos(theta3)*cos(theta6)*sin(theta4) - cos(theta6)*sin(theta2)*sin(theta3)*sin(theta4) - cos(theta2)*sin(theta3)*sin(theta5)*sin(theta6) - cos(theta3)*sin(theta2)*sin(theta5)*sin(theta6) + theta4*cos(theta2)*cos(theta3)*cos(theta4)*cos(theta6) - theta2*cos(theta2)*cos(theta6)*sin(theta3)*sin(theta4) - theta2*cos(theta3)*cos(theta6)*sin(theta2)*sin(theta4) - theta2*cos(theta2)*cos(theta3)*sin(theta5)*sin(theta6) - theta3*cos(theta2)*cos(theta6)*sin(theta3)*sin(theta4) - theta3*cos(theta3)*cos(theta6)*sin(theta2)*sin(theta4) - theta3*cos(theta2)*cos(theta3)*sin(theta5)*sin(theta6) - theta4*cos(theta4)*cos(theta6)*sin(theta2)*sin(theta3) - theta5*cos(theta2)*cos(theta5)*sin(theta3)*sin(theta6) - theta5*cos(theta3)*cos(theta5)*sin(theta2)*sin(theta6) - theta6*cos(theta2)*cos(theta3)*sin(theta4)*sin(theta6) - theta6*cos(theta2)*cos(theta6)*sin(theta3)*sin(theta5) - theta6*cos(theta3)*cos(theta6)*sin(theta2)*sin(theta5) + theta2*sin(theta2)*sin(theta3)*sin(theta5)*sin(theta6) + theta3*sin(theta2)*sin(theta3)*sin(theta5)*sin(theta6) + theta6*sin(theta2)*sin(theta3)*sin(theta4)*sin(theta6) + cos(theta2)*cos(theta3)*cos(theta4)*cos(theta5)*sin(theta6) - cos(theta4)*cos(theta5)*sin(theta2)*sin(theta3)*sin(theta6) + theta6*cos(theta2)*cos(theta3)*cos(theta4)*cos(theta5)*cos(theta6) - theta2*cos(theta2)*cos(theta4)*cos(theta5)*sin(theta3)*sin(theta6) - theta2*cos(theta3)*cos(theta4)*cos(theta5)*sin(theta2)*sin(theta6) - theta3*cos(theta2)*cos(theta4)*cos(theta5)*sin(theta3)*sin(theta6) - theta3*cos(theta3)*cos(theta4)*cos(theta5)*sin(theta2)*sin(theta6) - theta4*cos(theta2)*cos(theta3)*cos(theta5)*sin(theta4)*sin(theta6) - theta5*cos(theta2)*cos(theta3)*cos(theta4)*sin(theta5)*sin(theta6) - theta6*cos(theta4)*cos(theta5)*cos(theta6)*sin(theta2)*sin(theta3) + theta4*cos(theta5)*sin(theta2)*sin(theta3)*sin(theta4)*sin(theta6) + theta5*cos(theta4)*sin(theta2)*sin(theta3)*sin(theta5)*sin(theta6);;\nJ[4][1]  = \tcos(theta4)*cos(theta6) - cos(theta5)*sin(theta4)*sin(theta6) - theta4*cos(theta6)*sin(theta4) - theta6*cos(theta4)*sin(theta6) - theta4*cos(theta4)*cos(theta5)*sin(theta6) - theta6*cos(theta5)*cos(theta6)*sin(theta4) + theta5*sin(theta4)*sin(theta5)*sin(theta6);;\nJ[4][2]  = \tcos(theta4)*cos(theta6) - cos(theta5)*sin(theta4)*sin(theta6) - theta4*cos(theta6)*sin(theta4) - theta6*cos(theta4)*sin(theta6) - theta4*cos(theta4)*cos(theta5)*sin(theta6) - theta6*cos(theta5)*cos(theta6)*sin(theta4) + theta5*sin(theta4)*sin(theta5)*sin(theta6);;\nJ[4][3]  = sin(theta5)*sin(theta6) + theta5*cos(theta5)*sin(theta6) + theta6*cos(theta6)*sin(theta5);;\nJ[4][4]  = cos(theta6) - theta6*sin(theta6);\nJ[4][5]  = \t0;\n\nJ[5][0]  = \ttheta2*cos(theta5)*sin(theta2)*sin(theta3) - cos(theta3)*cos(theta5)*sin(theta2) - theta2*cos(theta2)*cos(theta3)*cos(theta5) - theta3*cos(theta2)*cos(theta3)*cos(theta5) - cos(theta2)*cos(theta5)*sin(theta3) + theta3*cos(theta5)*sin(theta2)*sin(theta3) + theta5*cos(theta2)*sin(theta3)*sin(theta5) + theta5*cos(theta3)*sin(theta2)*sin(theta5) - cos(theta2)*cos(theta3)*cos(theta4)*sin(theta5) + cos(theta4)*sin(theta2)*sin(theta3)*sin(theta5) - theta5*cos(theta2)*cos(theta3)*cos(theta4)*cos(theta5) + theta2*cos(theta2)*cos(theta4)*sin(theta3)*sin(theta5) + theta2*cos(theta3)*cos(theta4)*sin(theta2)*sin(theta5) + theta3*cos(theta2)*cos(theta4)*sin(theta3)*sin(theta5) + theta3*cos(theta3)*cos(theta4)*sin(theta2)*sin(theta5) + theta4*cos(theta2)*cos(theta3)*sin(theta4)*sin(theta5) + theta5*cos(theta4)*cos(theta5)*sin(theta2)*sin(theta3) - theta4*sin(theta2)*sin(theta3)*sin(theta4)*sin(theta5);;\nJ[5][1]  = \tsin(theta4)*sin(theta5) + theta4*cos(theta4)*sin(theta5) + theta5*cos(theta5)*sin(theta4);;\nJ[5][2]  = \tsin(theta4)*sin(theta5) + theta4*cos(theta4)*sin(theta5) + theta5*cos(theta5)*sin(theta4);;\nJ[5][3]  = \tcos(theta5) - theta5*sin(theta5);\nJ[5][4]  = \t0\t;\nJ[5][5]  = \t1;"("theta"=w18) -> ("J"=w19:dbl[][])
    }
  }
  "J" <- w8
  n7 = call-poly <vilib>:"Inverse Matrix.vi"("Input Matrix"=w8) -> ("Inverse Matrix"=w9:T1)  [unwired: 1 in, 1 out]
  n8 = Transpose Matrix(1:w8) -> (0:w12:dbl[][])
  "JT" <- w12
  n9 = call-poly <vilib>:"Matrix To Array.vi"("Real Matrix"=w9) -> ("Real 2D Array"=→"J-":dbl[][])
  n10 = call-poly <vilib>:"Inverse Matrix.vi"("Input Matrix"=w12) -> ("Inverse Matrix"=w11:T1)  [unwired: 1 in, 1 out]
  n11 = call-poly <vilib>:"Matrix To Array.vi"("Real Matrix"=w11) -> ("Real 2D Array"=→"J-T":dbl[][])
